vi "ex2_moje.vi"() -> ()   [LabVIEW 2022 SP3]
uses:
  <vilib>/numeric/Random Number (Range) DBL.vi
panel:
  out "text from file":string
  in  "File path":path
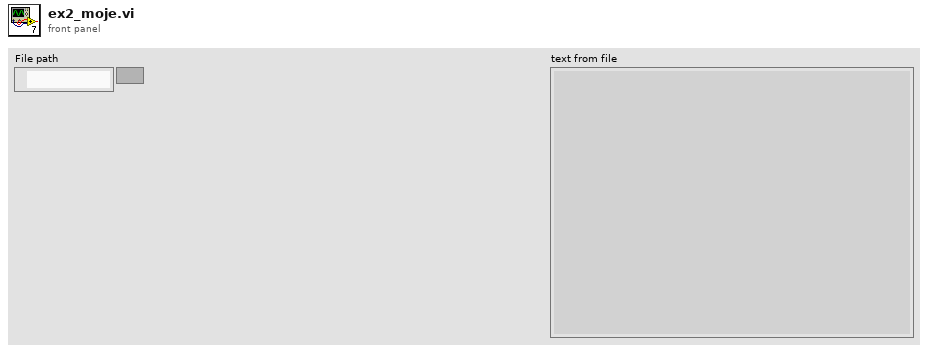
[diagram p1: front panel]
types:
  T1 = enum16{"open", "replace", "create", "open or create", "replace or create", "replace or create with confirmation"}
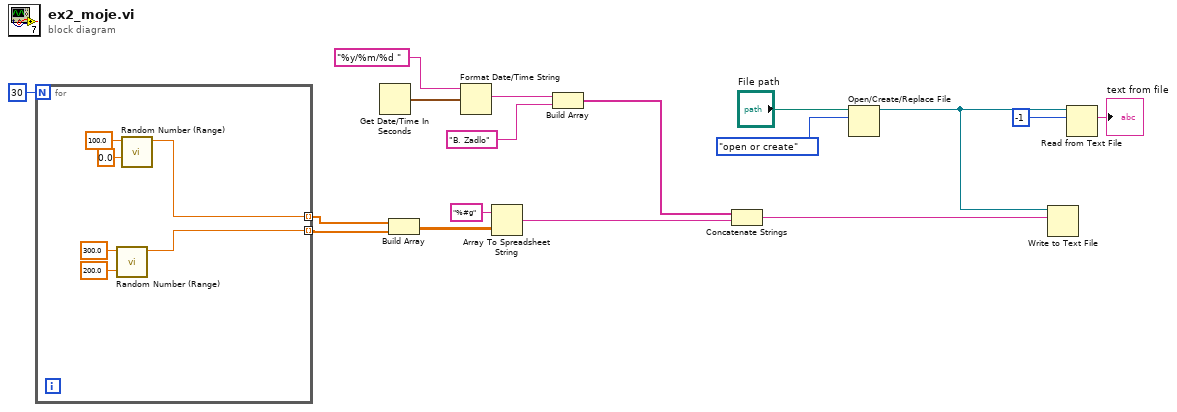
[diagram p0: block diagram]
diagram:
  n1 = for {
    N: 30 -> [_]
    tunnel: [w23] -> w17 mode=indexing
    tunnel: [w22] -> w16 mode=indexing
    n2 = call-poly <vilib>:"Random Number (Range).vi"("lower bound (0)"=200.0, "upper bound (100)"=300.0) -> ("number"=w22:dbl)  [unwired: 9 in]
    n3 = call-poly <vilib>:"Random Number (Range).vi"("lower bound (0)"=0.0, "upper bound (100)"=100.0) -> ("number"=w23:dbl)  [unwired: 9 in]
  }
  n4 = Get Date/Time In Seconds() -> (seconds since 1Jan1904=w13:timestamp)
  n5 = Build Array(w17, w16) -> (w9:dbl[][])
  n6 = Format Date/Time String(time format string (%c)="%y/%m/%d ", seconds (now)=w13) -> (date/time string=w11:string)  [unwired: 1 in]
  n7 = Array To Spreadsheet String(array=w9, 3:"%#g" ("format string")) -> (spreadsheet string=w6:string)  [unwired: 1 in]
  n8 = Build Array(w11, "B. Zadlo" ("element")) -> (w7:string[])
  n9 = Concatenate Strings(w7, w6) -> (w5:string)
  n10 = Open/Create/Replace File(file path (use dialog)="File path", operation (0:open)=T1."open or create") -> (refnum out=w2:refnum<file>)  [unwired: 4 in, 2 out]
  n11 = Write to Text File(file (use dialog)=w2, text=w5) -> ()  [unwired: 2 in, 3 out]
  n12 = Read from Text File(file (use dialog)=w2, count=-1) -> (text=→"text from file":string)  [unwired: 2 in, 3 out]
